vi "Power Read Array.vi"(8 "error in":errorcluster, 11 "Cycler in":refnum<class "Cycler.lvclass">) -> (0 "error out":errorcluster, 2 "Power SP":dbl[](array[numeric]), 3 "Cycler out":refnum<class "Cycler.lvclass">)   [LabVIEW 2023, in "Cycler.lvclass"]
uses:
  Cycler.lvclass
  Low Level Capabilities/Power/Power Setpoint/Power Setpoint.lvclass
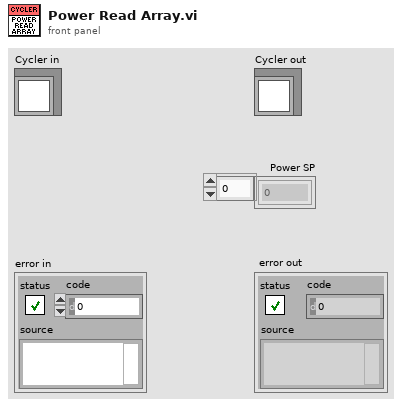
[diagram p1: front panel]
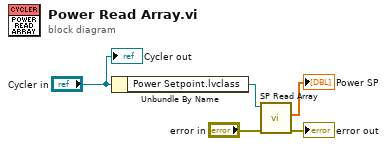
[diagram p0: block diagram]
diagram:
  n1 = Unbundle By Name("Cycler in") -> ("Power Setpoint.lvclass"=w2:refnum<class "Power Setpoint.lvclass">)
  n2 = call-dynamic "SP Read Array.vi"("error in"="error in", "Power Setpoint in"=w2) -> ("error out"=→"error out":errorcluster, "Power SP"=→"Power SP":dbl[])  [unwired: 6 in, 2 out]
  "Cycler out" <- "Cycler in"
